vi "AcquisitionProgram.vi"() -> ()   [LabVIEW 2019]
uses:
  <vilib>/Analysis/NI_AALPro.lvlib
  <vilib>/Analysis/2dsp.llb/Real FFT.vi
  <vilib>/Analysis/4window.llb/Gaussian Window (DBL).vi
panel:
  out "Spectrum":cluster{"Array":dbl[], "Array":dbl[]}(graph)
  out "Windowed Interferogram":cluster{"Array":dbl[], "Array":dbl[]}(graph)
  out "deltaX":dbl
  in  "set 0 position":bool
  out "Interferogram":cluster{"Array":dbl[], "Array":dbl[]}(graph)
  in  "scan":bool
  out "systemList":string[](array[string])
  out "systemIndex":u32
  in  "POSITION":i32
  in  "FREQUENCY":i32
  in  "AMPLITUDE":i32
  in  "STEPS":i32
  in  "stop":bool
  in  "backward":bool
  in  "move to position":bool
  in  "forward":bool
  in  "exit":bool
  out "Error":errorcluster
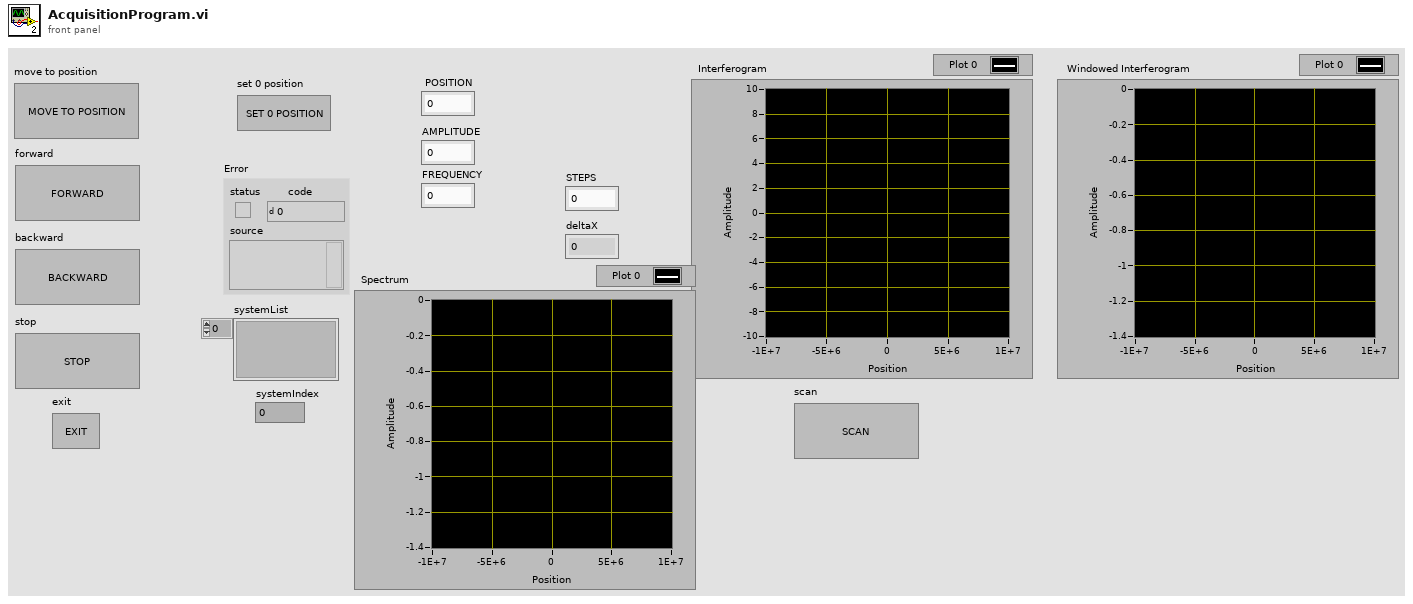
[diagram p1: front panel]
types:
  T1 = enum32{"SA_STOPPED_STATUS", "SA_STEPPING_STATUS", "SA_SCANNING_STATUS", "SA_HOLDING_STATUS", "SA_TARGET_STATUS", "SA_MOVE_DELAY_STATUS", "SA_CALIBRATING_STATUS", "SA_FINDING_REF_STATUS", "SA_OPENING_STATUS"}
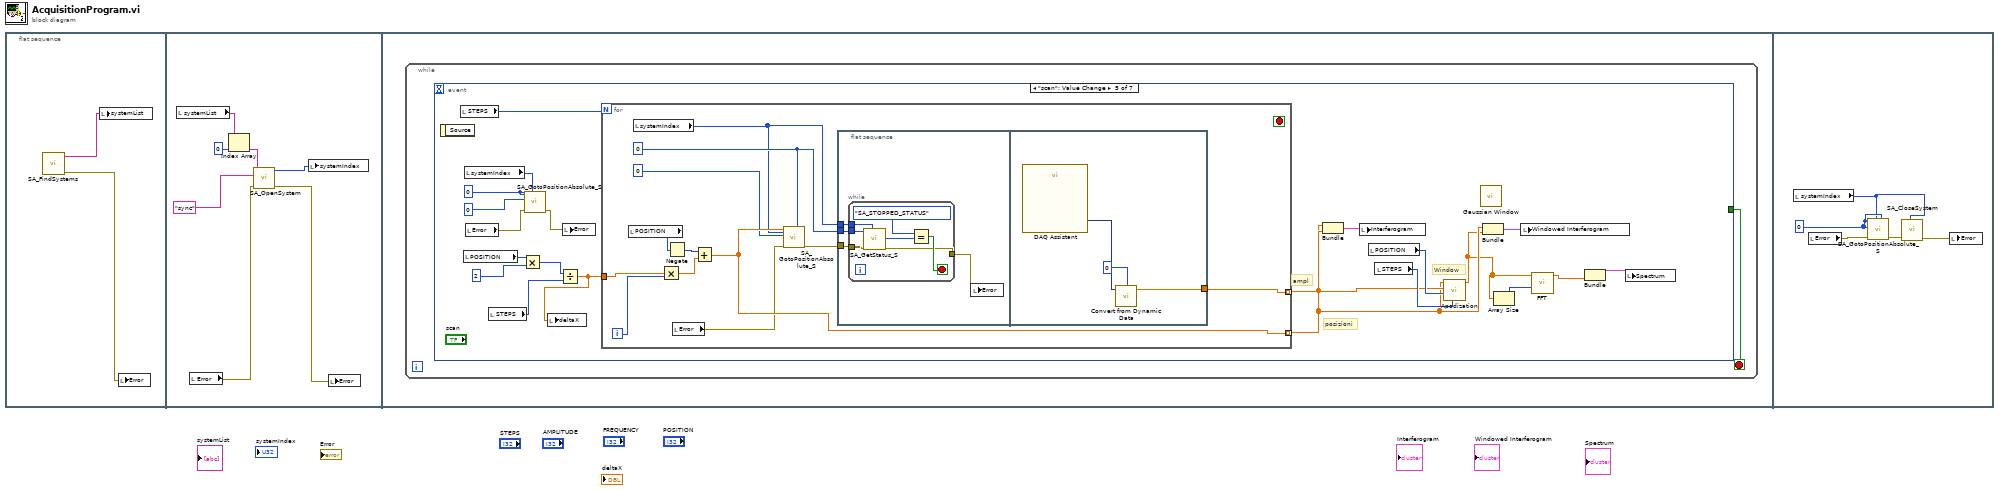
[diagram p0: block diagram]
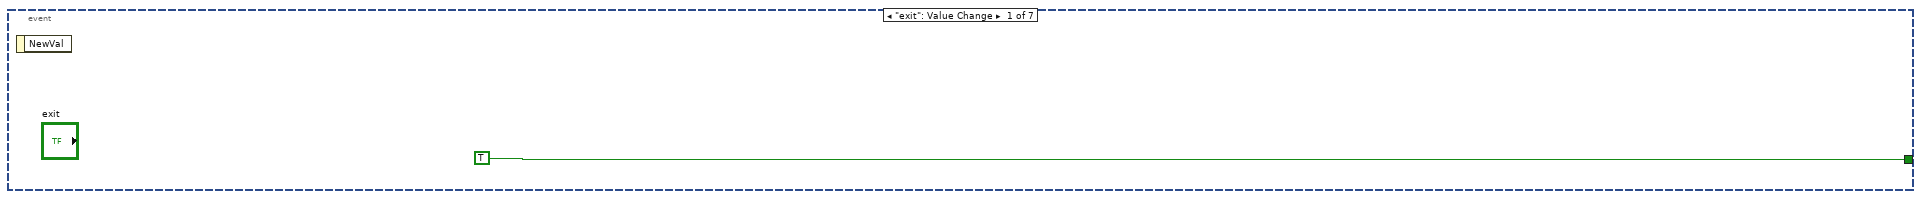
[diagram p2: hidden frame]
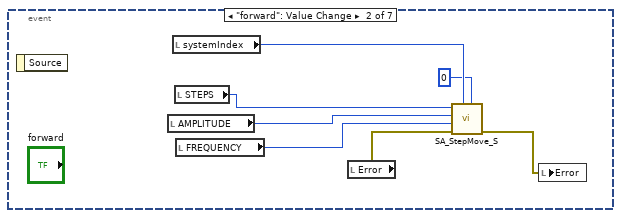
[diagram p3: hidden frame]
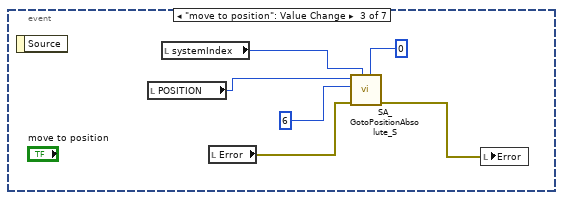
[diagram p4: hidden frame]
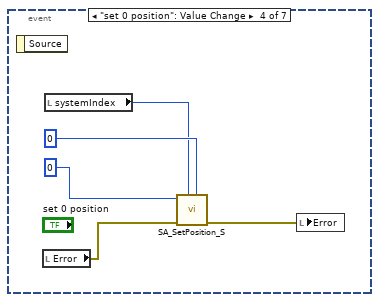
[diagram p5: hidden frame]
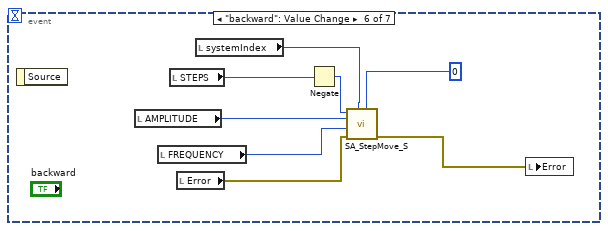
[diagram p6: hidden frame]
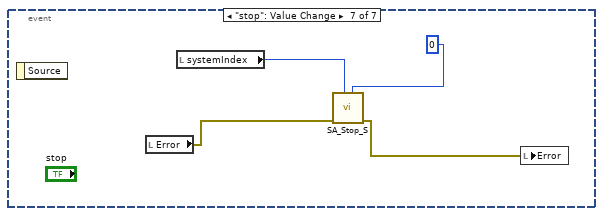
[diagram p7: hidden frame]
diagram:
  n1 = flat-sequence {
    frame #0 {
      n2 = call <vilib>:"SA_FindSystems.vi"() -> ("error out"=w2:errorcluster, "systemList"=w1:string[])  [unwired: 10 in]
      n3 = local write "systemList"(w1) -> ()
      n4 = local write "Error"(w2) -> ()
    }
    frame #1 {
      n5 = local read "systemList"() -> (w5:string[])
      n6 = local read "Error"() -> (w8:errorcluster)
      n7 = Index Array(array=w5, index=0) -> (element=w4:string)
      n8 = call <vilib>:"SA_OpenSystem.vi"("error in (no error)"=w8, "options"="sync", "systemLocator"=w4) -> ("error out"=w9:errorcluster, "systemIndexOut"=w7:u32)  [unwired: 7 in]
      n9 = local write "systemIndex"(w7) -> ()
      n10 = local write "Error"(w9) -> ()
    }
    frame #2 {
      n11 = while {
        stop <- w10 stop-if-true
        n12 = event shown="[4] \"scan\": Value Change" {
          selector: _ -> [_ _ _ _ _ _ _]
          dyn-events: _ -> [_ _ _ _ _ _ _]
          timeout: _ -> [_ _ _ _ _ _ _]
          tunnel: [TRUE _ _ _ _ _ _] -> w10
          event "exit": Value Change {
            n13 = event-data() -> ()  [unwired: 1 in, 1 out]
          }
          event "forward": Value Change {
            n14 = event-data() -> ()  [unwired: 1 in, 1 out]
            n15 = local read "AMPLITUDE"() -> (w17:i32)
            n16 = local read "systemIndex"() -> (w13:u32)
            n17 = local read "STEPS"() -> (w18:i32)
            n18 = local read "FREQUENCY"() -> (w16:i32)
            n19 = local read "Error"() -> (w14:errorcluster)
            n20 = call <vilib>:"SA_StepMove_S.vi"("channelIndex"=u32 0, "systemIndex"=w13, "error in (no error)"=w14, "frequency"=w16, "amplitude"=w17, "steps"=w18) -> ("error out"=w15:errorcluster)  [unwired: 5 in]
            n21 = local write "Error"(w15) -> ()
          }
          event "move to position": Value Change {
            n22 = event-data() -> ()  [unwired: 1 in, 1 out]
            n23 = local read "POSITION"() -> (w24:i32)
            n24 = local read "systemIndex"() -> (w22:u32)
            n25 = local read "Error"() -> (w21:errorcluster)
            n26 = call <vilib>:"SA_GotoPositionAbsolute_S.vi"("channelIndex"=u32 0, "systemIndex"=w22, "error in (no error)"=w21, "holdTime"=u32 6, "position"=w24) -> ("error out"=w20:errorcluster)  [unwired: 6 in]
            n27 = local write "Error"(w20) -> ()
          }
          event "set 0 position": Value Change {
            n28 = event-data() -> ()  [unwired: 1 in, 1 out]
            n29 = local read "Error"() -> (w29:errorcluster)
            n30 = local read "systemIndex"() -> (w25:u32)
            n31 = call <vilib>:"SA_SetPosition_S.vi"("channelIndex"=u32 0, "systemIndex"=w25, "error in (no error)"=w29, "position"=0) -> ("error out"=w28:errorcluster)  [unwired: 7 in]
            n32 = local write "Error"(w28) -> ()
          }
          event "scan": Value Change {
            w46 = u32 0 ("channelIndex")
            # "Window"
            # "ampl"
            # "posizioni"
            n33 = event-data() -> ()  [unwired: 1 in, 1 out]
            n34 = local read "STEPS"() -> (w50:i32)
            n35 = local read "POSITION"() -> (w43:i32)
            n36 = local read "systemIndex"() -> (w47:u32)
            n37 = local read "Error"() -> (w49:errorcluster)
            n38 = local read "STEPS"() -> (w44:i32)
            n39 = Multiply(x=w43, y=2 ("x")) -> (x*y=w42:i32)
            n40 = call <vilib>:"SA_GotoPositionAbsolute_S.vi"("channelIndex"=w46, "systemIndex"=w47, "error in (no error)"=w49, "holdTime"=u32 0, "position"=w46) -> ("error out"=w45:errorcluster)  [unwired: 6 in]
            n41 = Divide(x=w42, y=w44) -> (x/y=w41:dbl)
            n42 = local write "deltaX"(w41) -> ()
            n43 = local write "Error"(w45) -> ()
            n44 = for {
              N: w50 -> [_]
              tunnel: w41 -> [w62]
              tunnel: [w59] -> w35 mode=indexing
              tunnel: [w60] -> w36 mode=indexing
              i -> [w61]
              stop <- _ stop-if-true
              w56 = u32 0 ("channelIndex")
              n45 = local read "POSITION"() -> (w51:i32)
              n46 = local read "systemIndex"() -> (w55:u32)
              n47 = Multiply(x=w62, y=w61) -> (x*y=w53:dbl)
              n48 = Negate(x=w51) -> (-x=w52:i32)
              n49 = local read "Error"() -> (w58:errorcluster)
              n50 = Add(x=w52, y=w53) -> (x+y=w59:dbl)
              n51 = call <vilib>:"SA_GotoPositionAbsolute_S.vi"("channelIndex"=w56, "systemIndex"=w55, "error in (no error)"=w58, "holdTime"=u32 0, "position"=w59) -> ("error out"=w54:errorcluster)  [unwired: 6 in]
              n52 = flat-sequence {
                tunnel: w56 -> [w66]
                tunnel: w55 -> [w65]
                tunnel: w54 -> [w64]
                tunnel: [w75] -> w60
                frame #0 {
                  n53 = while {
                    tunnel: w66 -> [w71]
                    tunnel: w65 -> [w70]
                    tunnel: w64 -> [w69]
                    tunnel: [w67] -> w63
                    stop <- w72 stop-if-true
                    n54 = call <vilib>:"SA_GetStatus_S.vi"("channelIndex"=w71, "systemIndex"=w70, "error in (no error)"=w69) -> ("error out"=w67:errorcluster, "status"=w68:T1)  [unwired: 7 in]
                    n55 = Equal?(x=T1."SA_STOPPED_STATUS", y=w68) -> (x = y?=w72:bool)
                  }
                  n56 = local write "Error"(w63) -> ()
                }
                frame #1 {
                  n57 = call "DAQ Assistant"() -> ("data"=w74:dynamicdata)  [unwired: 17 in, 2 out]
                  n58 = call "Convert from Dynamic Data"("Dynamic Data Type"=w74, "Channel"=0) -> ("Scalar"=w75:dbl)  [unwired: 2 in]
                }
              }
            }
            n59 = Bundle(w35, w36) -> (w39:cluster{dbl[], dbl[]})  [unwired: 1 in]
            n60 = local write "Interferogram"(w39) -> ()
            n61 = local read "POSITION"() -> (w38:i32)
            n62 = local read "STEPS"() -> (w37:i32)
            n63 = call "Apodization.vi"("STEPS"=w37, "POSITION"=w38, "y"=w36, "x"=w35) -> ("Apodized_y"=w32:dbl[])  [unwired: 7 in]
            n64 = call-poly <vilib>:"Gaussian Window.vi"() -> ()  [unwired: 10 in, 2 out]
            n65 = Bundle(w35, "Apodized_y"=w32) -> (w34:cluster{dbl[], "Apodized_y":dbl[]})  [unwired: 1 in]
            n66 = Array Size(array=w32) -> (size(s)=w33:i32)
            n67 = local write "Windowed Interferogram"(w34) -> ()
            n68 = call-poly <vilib>:"FFT.vi"("FFT size"=w33, "X"=w32) -> ("FFT {X}"=w30:cdb[])  [unwired: 8 in, 1 out]
            n69 = Bundle("FFT {X}"=w30) -> (w31:cluster{void, "FFT {X}":cdb[]})  [unwired: 2 in]
            n70 = local write "Spectrum"(w31) -> ()
          }
          event "backward": Value Change {
            n71 = event-data() -> ()  [unwired: 1 in, 1 out]
            n72 = local read "AMPLITUDE"() -> (w79:i32)
            n73 = local read "FREQUENCY"() -> (w84:i32)
            n74 = local read "STEPS"() -> (w78:i32)
            n75 = local read "Error"() -> (w83:errorcluster)
            n76 = local read "systemIndex"() -> (w81:u32)
            n77 = Negate(x=w78) -> (-x=w77:i32)
            n78 = call <vilib>:"SA_StepMove_S.vi"("channelIndex"=u32 0, "systemIndex"=w81, "error in (no error)"=w83, "frequency"=w84, "amplitude"=w79, "steps"=w77) -> ("error out"=w82:errorcluster)  [unwired: 5 in]
            n79 = local write "Error"(w82) -> ()
          }
          event "stop": Value Change {
            n80 = event-data() -> ()  [unwired: 1 in, 1 out]
            n81 = local read "Error"() -> (w87:errorcluster)
            n82 = local read "systemIndex"() -> (w85:u32)
            n83 = call <vilib>:"SA_Stop_S.vi"("channelIndex"=0, "systemIndex"=w85, "error in (no error)"=w87) -> ("error out"=w88:errorcluster)  [unwired: 8 in]
            n84 = local write "Error"(w88) -> ()
          }
        }
      }
    }
    frame #3 {
      w90 = u32 0 ("holdTime")
      n85 = local read "systemIndex"() -> (w89:u32)
      n86 = local read "Error"() -> (w92:errorcluster)
      n87 = call <vilib>:"SA_GotoPositionAbsolute_S.vi"("channelIndex"=w90, "systemIndex"=w89, "error in (no error)"=w92, "holdTime"=w90, "position"=w90) -> ("error out"=w91:errorcluster)  [unwired: 6 in]
      n88 = call <vilib>:"SA_CloseSystem.vi"("systemIndex"=w89, "error in (no error)"=w91) -> ("error out"=w93:errorcluster)  [unwired: 9 in]
      n89 = local write "Error"(w93) -> ()
    }
  }
